vi "get channels.vi"(11 "module configuration in":refnum<class "TBM module configuration.lvclass">) -> (2 "channels":refnum<class "TBM channel.lvclass">[](array[class]), 3 "module configuration out":refnum<class "TBM module configuration.lvclass">)   [LabVIEW 2013, in "TBM module configuration.lvclass"]
doc: "Returns all channels used by a module."
uses:
  TBM module configuration.lvclass
  channel/TBM channel.lvclass
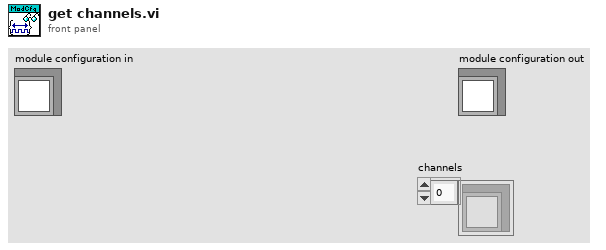
[diagram p1: front panel]
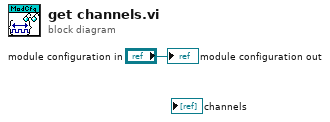
[diagram p0: block diagram]
diagram:
  "module configuration out" <- "module configuration in"
